vi "Get Existing Table Info.vi"(8 "error in (no error)":errorcluster, 10 "Table Name":string, 11 "Database in":refnum<class "Database Platform.lvclass">) -> (0 "error out":errorcluster, 2 "Column Info":T1, 3 "Database out":refnum<class "Database Platform.lvclass">)   [LabVIEW 2020, in "Conditu2.lvlib" / "Database Platform.lvclass"]
uses:
  Database Platform.lvclass
  Column Info.ctl
  Columns/Type/Type.lvclass
  Conditu2.lvlib
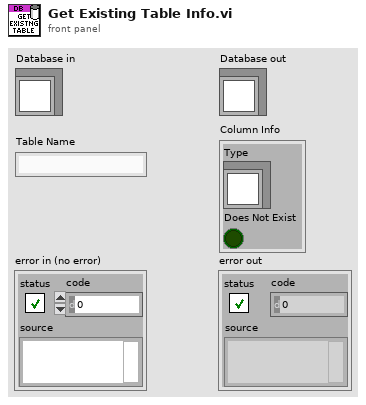
[diagram p1: front panel]
types:
  T1 = typedef "Conditu2.lvlib/Column Info.ctl" = cluster{"Type":refnum<class "Type.lvclass">, "Does Not Exist":bool}
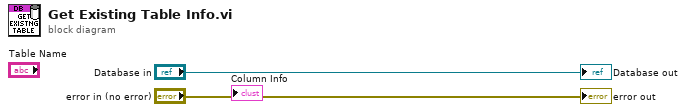
[diagram p0: block diagram]
diagram:
  "error out" <- "error in (no error)"
  "Database out" <- "Database in"
